vi "Add Component Configuration.vi"(7 "component name":string, 8 "error in (no error)":errorcluster, 10 "Configuration":refnum<class "Configuration.lvclass">, 11 "component settings in":T1[](array[typedef])) -> (0 "error out":errorcluster, 1 "no settings?":bool, 3 "component settings out":T1[](array[typedef]))   [LabVIEW 2017, in "DSF Core.lvlib"]
uses:
  DSF Core.lvlib
  Typedefs/DSF Settings Info.ctl
  Typedefs/DSF Version Info.ctl
  Classes/Configuration/Configuration.lvclass
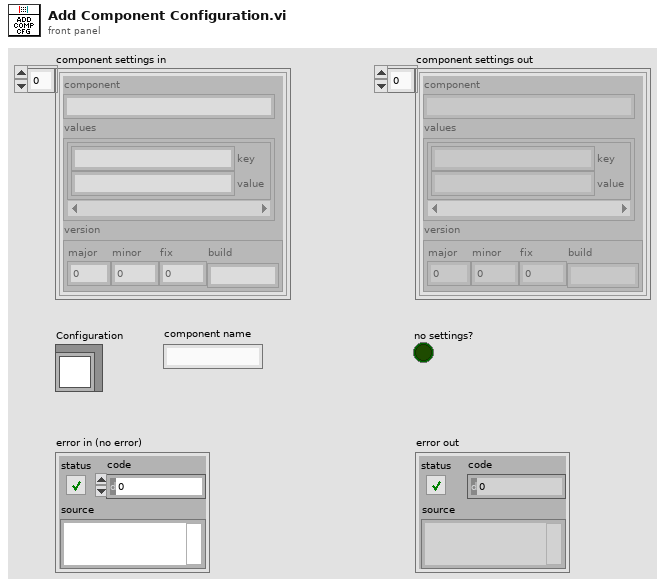
[diagram p1: front panel]
types:
  T1 = typedef "DSF Core.lvlib/DSF Settings Info.ctl" = cluster{"component":string, "values":cluster{"key":string, "value":string}[], "version":T2}
  T2 = typedef "DSF Core.lvlib/DSF Version Info.ctl" = cluster{"major":u32, "minor":u32, "fix":u32, "build":string}
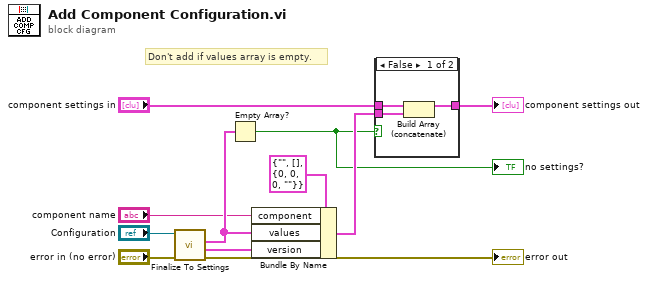
[diagram p0: block diagram]
diagram:
  # "Don't add if values array is empty."
  n1 = call-dynamic "Finalize To Settings.vi"("error in (no error)"="error in (no error)", "Configuration in"="Configuration") -> ("error out"=→"error out":errorcluster, "settings version"=w8:T2, "settings"=w5:cluster{"key":string, "value":string}[])  [unwired: 6 in, 1 out]
  n2 = Empty Array?(array=w5) -> (empty?=w2:bool)
  "no settings?" <- w2
  n3 = Bundle By Name(cluster=T1 {"component"="", "values"=[], "version"={"major"=0, "minor"=0, "fix"=0, "build"=""}} ("component settings out"), "component"="component name", "values"=w5, "version"=w8) -> (w4:T1)
  n4 = case shown="False" w2 {
    tunnel: "component settings in" -> [w14 w15]
    tunnel: w4 -> [w13 _]
    tunnel: [w12 w15] -> w3
    frame False {
      n5 = Build Array (concatenate)(w14, w13) -> (w12:T1[])
    }
    frame True {
    }
  }
  "component settings out" <- w3
